vi "T_Image_main03.vi"() -> ()   [LabVIEW 2018]
doc: "This example performs writes and reads on a serial port, as directed by the user. You can press the Write and Read buttons, and change the Read Count, while the example is running.\n\nThe parameters set for the serial port must match the parameters of the connected instrument or device. In this example, the Read Count parameter specifies the number of bytes that the serial port reads. If there were more bytes at the port than the specified number, those bytes would not be read. If there were less bytes at the port than the specified number, you would receive a timeout error.\n\nThis example expands upon the flow control options for XON and XOFF, allowing the user to choose those control characters. Also, the user can enable or disable a termination character. Some devices require a termination character in order to identify the end of command strings. Some devices send a termination character to signify the end of data to be read. This example shows how you can end the Read operation once a termination character is detected in the buffer and/or append a termination character at the end of the Write data."
uses:
  <vilib>/userdefined/High Color/IMAQdx.ctl
  <vilib>/Math Plots/3D Math Plots/3D Surface/3D Surface XCtrl/3D Surface.xctl
  <vilib>/Instr/_visa.llb/VISA Configure Serial Port (Instr).vi
  <vilib>/Math Plots/3D Math Plots/3D Surface/3D Surface Datatype/Public/Plot Helper (Matrix).vi
  <vilib>/vision/driver/NI_Vision_Acquisition_Software.lvlib
  <vilib>/vision/NI_Vision_Development_Module.lvlib
  <vilib>/Math Plots/3D Math Plots/3D Surface/3D Surface Datatype/3D Surface Datatype.lvclass
panel:
  in  "탭 컨트롤":enum32{"  2D ", "  3D "}(tab)
  out "Temperature":dbl[][](graph)
  in  "폭":dbl=10.0
  in  "중심":dbl=35.0
  out "3D Surface 2":refnum<class "3D Plot Datatype.lvclass">[](xcontrol) caption="3D 표면"
  in  "길이":i32=1
  in  "인덱스 (열)":i32
  out "최대":dbl
  out "웨이브폼 차트":dbl(graph)
  in  "열 화상 촬영":path
  in  "stop 4":bool
  in  "stop 3":bool
  out "Cam  2":T1(plugin-control)
  in  "Camera":T2="cam5"
  in  "stop":bool
  in  "stop 2":bool
  in  "VISA resource name":refnum<visa-resource-name>="COM6"
  in  "Stop":bool
  # "열화상 카메라"
  # "(Programmed by Hello Mr. Ko)"
  # "℃"
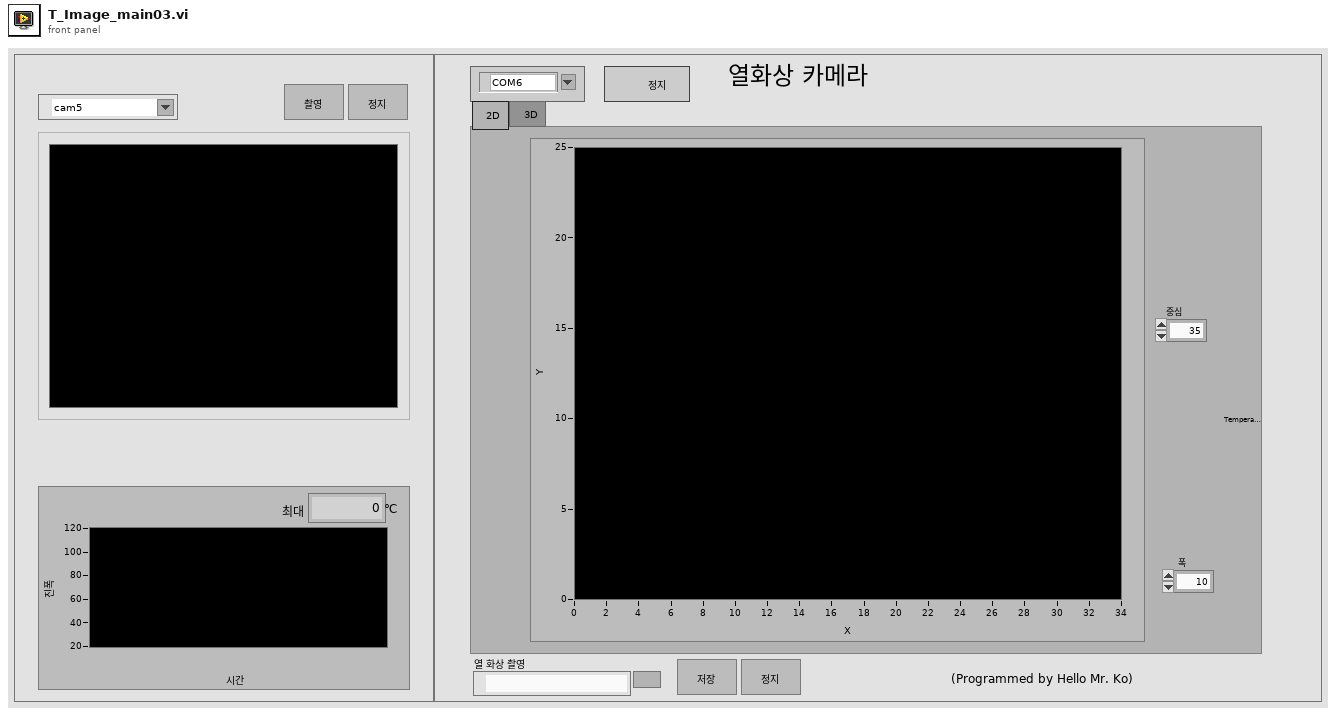
[diagram p1: front panel]
types:
  T1 = typedef "IMAQ Image.ctl" = refnum<image>
  T2 = typedef "IMAQdx.ctl" = refnum<k21>
  T3 = typedef "Image Type" = u32
  T4 = typedef "IMAQ AVI2 Refnum.ctl" = refnum<k20>
  T5 = typedef "imagedata.ctl" = cluster{"image type":i32, "image depth":i32, "image":u8[], "mask":u8[], "colors":u32[], "Rectangle":cluster{"left":i16, "top":i16, "right":i16, "bottom":i16}}
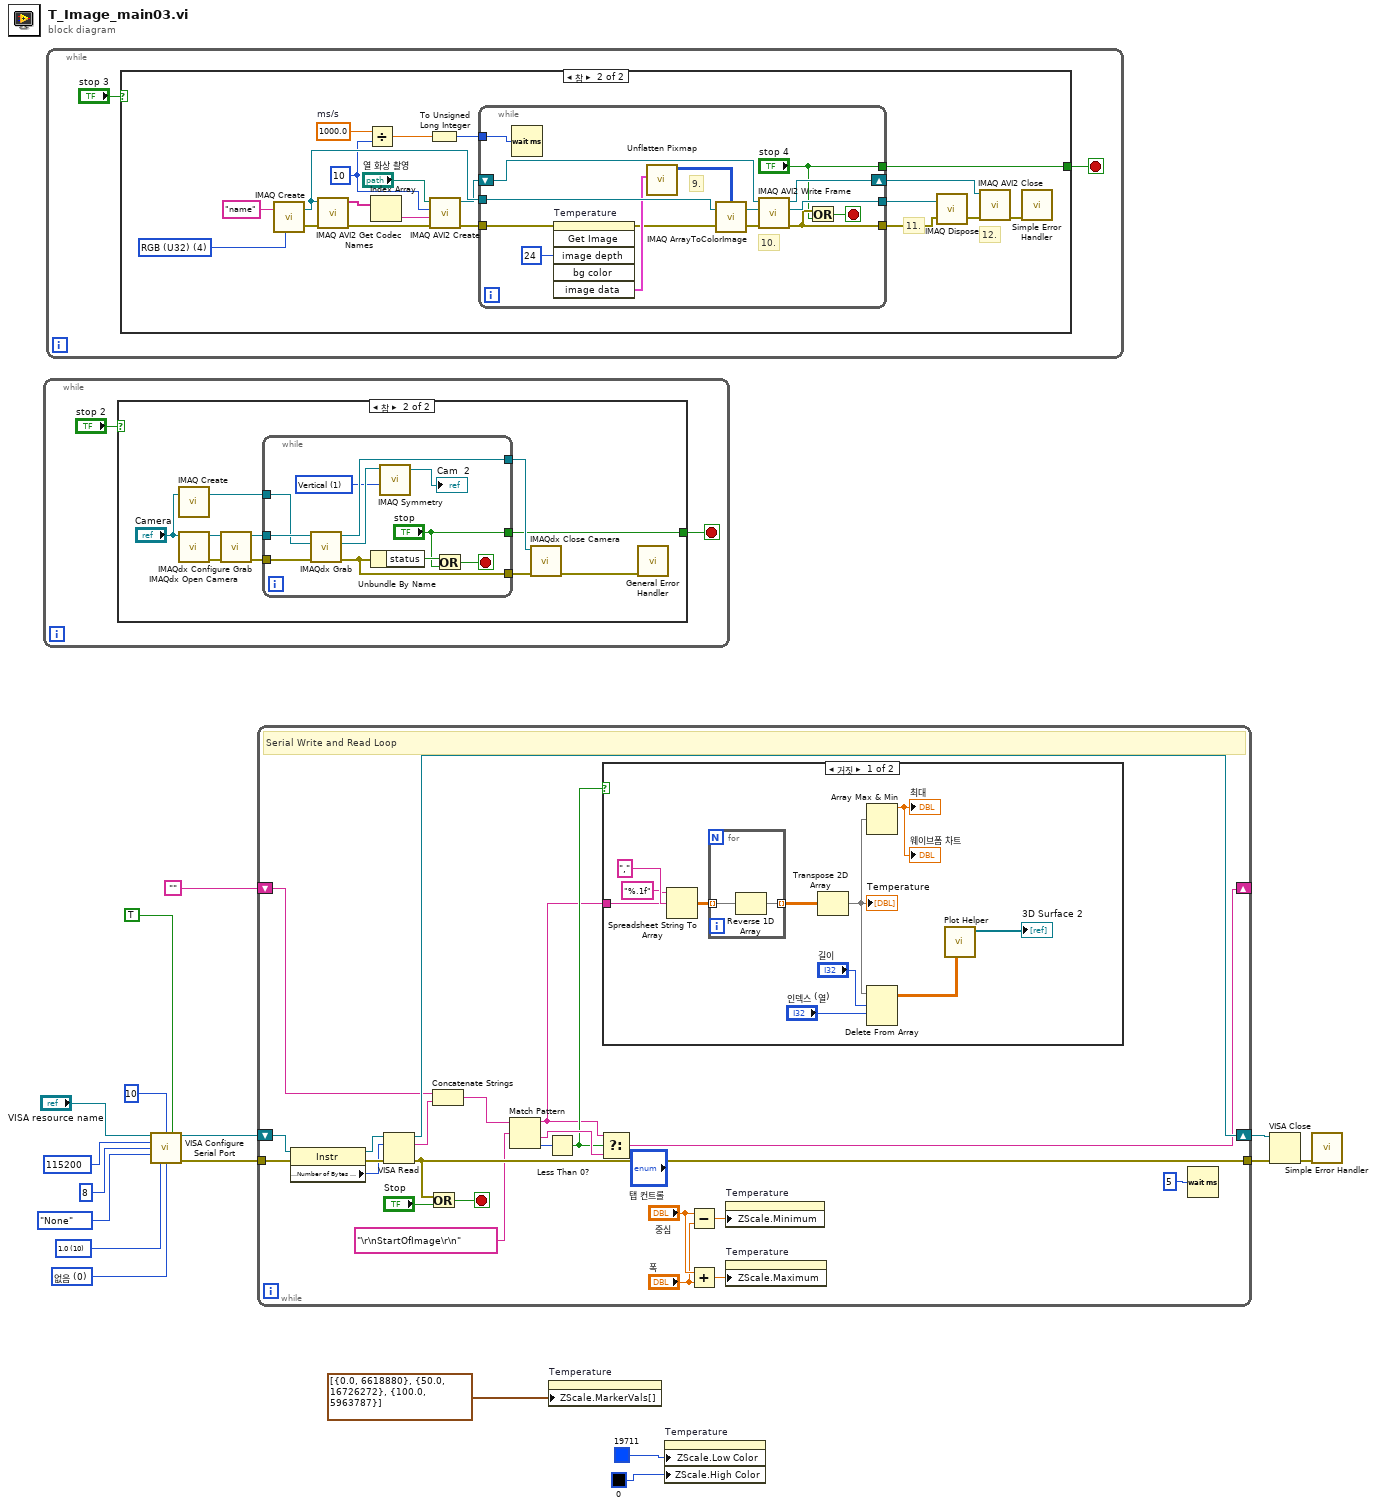
[diagram p0: block diagram]
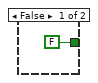
[diagram p2: hidden frame]
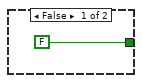
[diagram p3: hidden frame]
diagram:
  w4 = u16 0 items=["없음", "XON/XOFF", "RTS/CTS", "XON/XOFF & RTS/CTS", "DTR/DSR", "XON/XOFF & DTR/DSR"] ("flow control (0:none)")
  w5 = u16 10 items=["1.0"=10, "1.5"=15, "2.0"=20] ("stop bits (10: 1 bit)")
  n1 = while {
    stop <- w18 stop-if-true
    n2 = case shown="참" "stop 2" {
      tunnel: [FALSE ("stop") w21] -> w18
      frame False {
      }
      frame True {
        n3 = call "IMAQ Create"("Image Name"="Camera") -> ("New Image"=w30:T1)  [unwired: 3 in, 2 out]
        n4 = call <vilib>:"IMAQdx Open Camera.vi"("Session In"="Camera") -> ("error out"=w24:errorcluster, "Session Out"=w26:T2)  [unwired: 2 in, 7 out]
        n5 = call <vilib>:"IMAQdx Configure Grab.vi"("error in"=w24, "Session In"=w26) -> ("error out"=w22:errorcluster, "Session Out"=w23:T2)  [unwired: 1 in, 7 out]
        n6 = while {
          tunnel: [w36] -> w29
          tunnel: w22 -> [w38]
          tunnel: w23 -> [w39]
          tunnel: [w35] -> w28
          tunnel: w30 -> [w37]
          tunnel: ["stop"] -> w21
          stop <- w41 stop-if-true
          w31 = u32 1 items=["Horizontal", "Vertical", "Central", "1st Diagonal", "2nd Diagonal"] ("Type of Symmetry")
          n7 = call <vilib>:"IMAQdx Grab.vi"("error in"=w38, "Image In"=w37, "Session In"=w39) -> ("error out"=w35:errorcluster, "Image Out"=w33:T1, "Session Out"=w36:T2)  [unwired: 5 in, 1 out]
          n8 = Unbundle By Name(w35) -> ("status"=w40:bool)
          n9 = call "IMAQ Symmetry"("Type of Symmetry"=w31, "Image Src"=w33) -> ("Image Dst Out"=→"Cam  2":T1)  [unwired: 3 in, 1 out]
          n10 = Or(x=w40, y="stop") -> (x .or. y?=w41:bool)
        }
        n11 = call <vilib>:"IMAQdx Close Camera.vi"("error in"=w28, "Session In"=w29) -> ("error out"=w27:errorcluster)  [unwired: 9 out]
        n12 = call <vilib>:"General Error Handler.vi"("error in (no error)"=w27) -> ()  [unwired: 2 in, 13 out]
      }
    }
  }
  n13 = while {
    stop <- w42 stop-if-true
    n14 = case shown="참" "stop 3" {
      tunnel: [FALSE ("stop") w46] -> w42
      frame False {
      }
      frame True {
        w45 = u32 10 ("Frames/ Per Second")
        w49 = 1000.0  # ms/s
        w47 = T3 4 items=["Grayscale (U8)", "Grayscale (I16)", "Grayscale (SGL)", "Complex (CSG)", "RGB (U32)", "HSL (U32)", "RGB (U64)", "Grayscale (U16)"] ("Image Type")
        # "12."
        # "11."
        n15 = call "IMAQ Create"("Image Name"="name", "Image Type"=w47) -> ("New Image"=w59:T1, "error out"=w58:errorcluster)  [unwired: 3 in]
        n16 = call "IMAQ AVI2 Get Codec Names"("error in (no error)"=w58, "Image"=w59) -> ("error out"=w57:errorcluster, "Codec Names"=w61:string[])  [unwired: 8 in]
        n17 = Divide(x=w49, y=w45) -> (x/y=w63:dbl)
        n18 = Index Array(array=w61) -> (element=w62:string)  [unwired: 1 in]
        n19 = To Unsigned Long Integer(number=w63) -> (unsigned 32bit integer=w64:u32)
        n20 = call "IMAQ AVI2 Create"("error in (no error)"=w57, "Codec"=w62, "Frames Per Second"=w45, "AVI Path"="열 화상 촬영") -> ("error out"=w60:errorcluster, "AVI Refnum"=w56:T4)  [unwired: 6 in]
        n21 = while {
          tunnel: w59 -> [w73]
          tunnel: w60 -> [w67]
          tunnel: [w77] -> w50
          tunnel: [w74] -> w51
          shift-right: [w78] -> w52
          shift-left: w56 -> [w79]
          tunnel: w64 -> [w76]
          tunnel: ["stop 4"] -> w46
          stop <- w75 stop-if-true
          # "10."
          # "9."
          n22 = Wait (ms)(milliseconds to wait=w76) -> ()  [unwired: 1 out]
          n23 = invoke on="Temperature" class="IntGraph (엄격한)" method="Get Image"(error in=w67, "image depth"=24 ("Image Depth")) -> (error out=w66:errorcluster, "image data"=w68:T5)  [unwired: 4 in, 4 out]
          n24 = call <vilib>:"Unflatten Pixmap.vi"("image data"=w68) -> ("24-bit pixmap"=w70:u32[][])  [unwired: 4 in, 6 out]
          n25 = call "IMAQ ArrayToColorImage"("Image Pixels (U32)"=w70, "Image"=w73, "error in (no error)"=w66) -> ("Image Out"=w72:T1, "error out"=w71:errorcluster)  [unwired: 2 in]
          n26 = call "IMAQ AVI2 Write Frame"("error in (no error)"=w71, "Image"=w72, "AVI Refnum"=w79) -> ("error out"=w74:errorcluster, "Image Out (duplicate)"=w77:T1, "AVI Refnum (duplicate)"=w78:T4)  [unwired: 6 in]
          n27 = Or(x=w74, y="stop 4") -> (x .or. y?=w75:bool)
        }
        n28 = call "IMAQ Dispose"("Image"=w50, "error in (no error)"=w51) -> ("error out"=w53:errorcluster)  [unwired: 4 in]
        n29 = call "IMAQ AVI2 Close"("error in (no error)"=w53, "AVI Refnum"=w52) -> ("error out"=w54:errorcluster)  [unwired: 9 in]
        n30 = call <vilib>:"Simple Error Handler.vi"("error in (no error)"=w54) -> ()  [unwired: 4 in, 5 out]
      }
    }
  }
  n31 = call-poly "VISA Configure Serial Port"("VISA resource name"="VISA resource name", "termination char\n(0xA = '\\n' = LF)"=u8 10 ("Termination Character"), "Enable Termination\nChar (T)"=TRUE ("End Read on Termination Character?"), "baud rate (9600)"=u32 115200, "data bits (8)"=u16 8, "parity (0:none)"=enum16{"None", "Odd", "Even", "Mark", "Space"}."None", "stop bits (10: 1 bit)"=w5, "flow control (0:none)"=w4) -> ("VISA resource name out"=w11:refnum<visa-resource-name>, "error out"=w10:errorcluster)  [unwired: 2 in, 4 out]
  n32 = while {
    shift-right: [w97] -> w13
    shift-left: w11 -> [w99]
    tunnel: w10 -> [w95]
    tunnel: [w91] -> w14
    shift-right: [w84] -> _
    shift-left: "" -> [w93]
    stop <- w101 stop-if-true
    # "Serial Write and Read Loop"
    n33 = property class="Instr"(reference=w99, error in=w95) -> (reference out=w98:refnum<visa-resource-name>, error out=w96:errorcluster, "Serial Settings:Number of Bytes at Serial Port"=w94:u32)
    n34 = VISA Read(VISA resource name=w98, byte count=w94, error in (no error)=w96) -> (VISA resource name out=w97:refnum<visa-resource-name>, read buffer=w92:string, error out=w91:errorcluster)  [unwired: 1 out]
    n35 = Or(x=w91, y="Stop") -> (x .or. y?=w101:bool)
    n36 = Concatenate Strings(w93, w92) -> (w89:string)
    n37 = Match Pattern(string=w89, regular expression="\r\nStartOfImage\r\n") -> (before substring=w85:string, after substring=w87:string, offset past match=w88:i32)  [unwired: 1 in, 1 out]
    n38 = Less Than 0?(x=w88) -> (x < 0?=w86:bool)
    n39 = Select(t=w85, s=w86, f=w87) -> (s? t:f=w84:string)
    n40 = case shown="거짓" w86 {
      tunnel: w85 -> [w112 _]
      frame False {
        n41 = Spreadsheet String To Array(delimiter (Tab)=",", format string="%.1f", spreadsheet string=w112) -> (array=w110:dbl[][])  [unwired: 1 in]
        n42 = for {
          tunnel: w110 -> [w115] mode=indexing
          tunnel: [w114] -> w109 mode=indexing
          n43 = Reverse 1D Array(array=w115) -> (reversed array=w114:dbl[])
        }
        n44 = Transpose 2D Array(2D array=w109) -> (transposed array=w103:dbl[][])
        "Temperature" <- w103
        n45 = Array Max & Min(array=w103) -> (max value=→"최대" →"웨이브폼 차트":dbl)  [unwired: 3 out]
        n46 = Delete From Array(array=w103, length="길이", index (row)="인덱스 (열)") -> (array with subset deleted=w106:dbl[][])  [unwired: 1 in, 1 out]
        n47 = call-poly <vilib>:"Plot Helper.vi"("z matrix"=w106) -> ("3D Plot lvclass Array out"=→"3D Surface 2":refnum<class "3D Plot Datatype.lvclass">[])  [unwired: 5 in, 5 out]
      }
      frame True {
      }
    }
    n48 = Subtract(x="중심", y="폭") -> (x-y=w80:dbl)
    n49 = Add(x="중심", y="폭") -> (x+y=w83:dbl)
    n50 = property on="Temperature" class="IntGraph (엄격한)"("ZScale.Minimum"=w80) -> ()  [unwired: 2 in, 2 out]
    n51 = property on="Temperature" class="IntGraph (엄격한)"("ZScale.Maximum"=w83) -> ()  [unwired: 2 in, 2 out]
    n52 = Wait (ms)(milliseconds to wait=u32 5) -> ()  [unwired: 1 out]
  }
  n53 = property on="Temperature" class="IntGraph (엄격한)"("ZScale.MarkerVals[]"=cluster{dbl, u32}[] [{0.0, 6618880}, {50.0, 16726272}, {100.0, 5963787}] ("Z 스케일.마커 값[]")) -> ()  [unwired: 2 in, 2 out]
  n54 = property on="Temperature" class="IntGraph (엄격한)"("ZScale.Low Color"=u32 19711, "ZScale.High Color"=u32 0) -> ()  [unwired: 2 in, 2 out]
  n55 = VISA Close(VISA resource name=w13, error in (no error)=w14) -> (error out=w15:errorcluster)
  n56 = call <vilib>:"Simple Error Handler.vi"("error in (no error)"=w15) -> ()  [unwired: 1 in, 8 out]
